vi "Launch Listener.vi"(8 "error in (no error)":errorcluster, 9 "Endpoint":refnum<class "Endpoint.lvclass">, 10 "Listener Notifier":T1, 11 "Listener":refnum<k5>) -> (0 "error out":errorcluster)   [LabVIEW 2020, in "Stream-TCP.lvlib" / "TCP Client.lvclass"]
uses:
  TCP Client.lvclass
  Listener Notifier.ctl
  Listener Status.ctl
  lv-stream/stream/Endpoint/Endpoint.lvclass
  Listener Async.vi
  Stream-TCP.lvlib
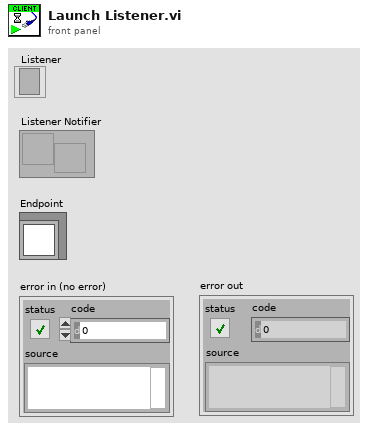
[diagram p1: front panel]
types:
  T1 = typedef "Stream-TCP.lvlib/Listener Notifier.ctl" = refnum<notifier>
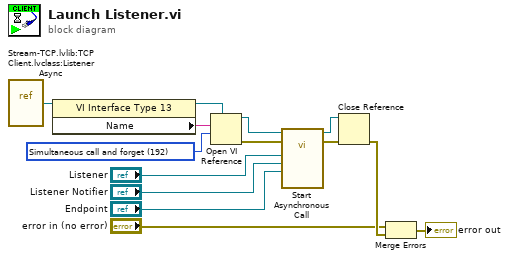
[diagram p0: block diagram]
diagram:
  w9 = 192 items=["Record modifications"=1, "Open templates for editing"=2, "Prompt user to save"=4, "Prepare for reentrant run"=8, "Prompt to find missing subVIs"=16, "Hide loading dialog box"=32, "Enable simultaneous calls"=64, "Prepare to call and forget"=128, "Simultaneous call and forget"=192, "Prepare to call and collect"=256, "Simultaneous call and collect"=320]
  n1 = vi-ref "Stream-TCP.lvlib:TCP Client.lvclass:Listener Async.vi"() -> (w7:refnum<vi>)
  n2 = property class="VI Interface Type 13"(reference=w7) -> (reference out=w10:refnum<vi>, "Name"=w8:string)  [unwired: 1 in, 1 out]
  n3 = Open VI Reference(type specifier VI Refnum (for type only)=w10, vi path=w8, options=w9) -> (vi reference=w12:refnum<vi>, error out=w11:errorcluster)  [unwired: 3 in]
  n4 = call-by-ref "Start Asynchronous Call"(reference=w12, error in=w11, "Endpoint"="Endpoint", "Listener Notifier"="Listener Notifier", "Listener"="Listener") -> (reference out=w14:refnum<vi>, error out=w13:errorcluster)  [unwired: 9 in]
  n5 = Close Reference(reference=w14, error in (no error)=w13) -> (error out=w3:errorcluster)
  n6 = Merge Errors("error in (no error)", w3) -> (→"error out":errorcluster)
